vi "f.vi"() -> ()   [LabVIEW 2018]
uses:
  <vilib>/regexp/Match Regular Expression.xnode
panel:
  out "Array":string[](array[string])
  in  "length (rest) 2":i32
  in  "offset (0) 2":i32
  out "substring 2":string
  in  "length (rest)":i32
  in  "offset (0)":i32
  out "substring":string
  in  "Stop":bool
  out "Input":string
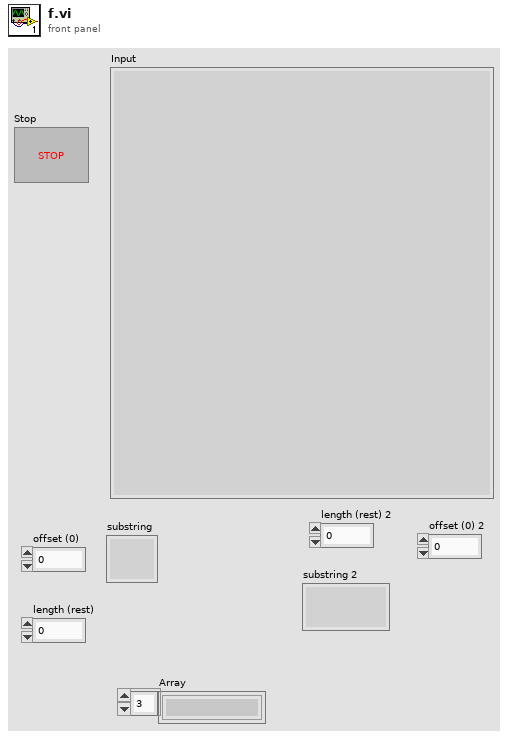
[diagram p1: front panel]
types:
  T1 = enum16{"open", "replace", "create", "open or create", "replace or create", "replace or create with confirmation"}
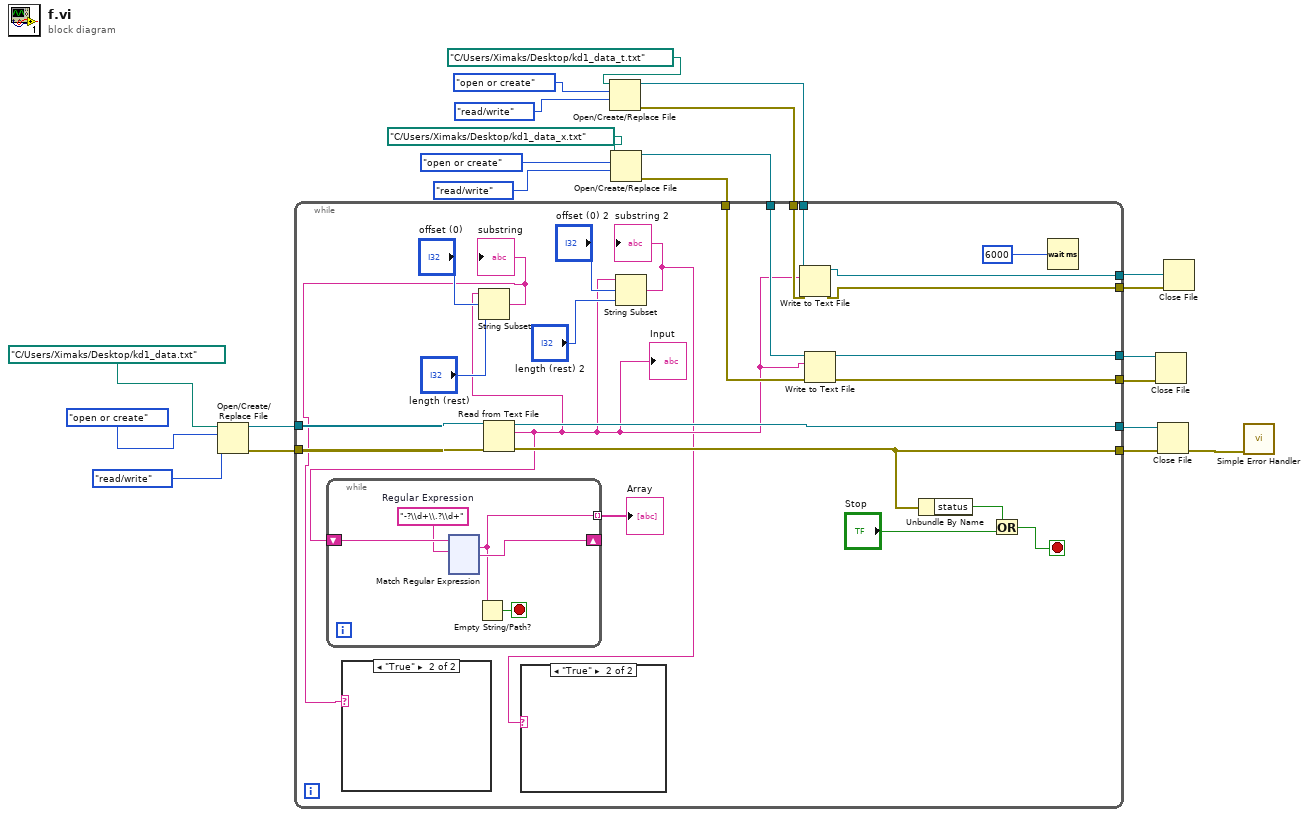
[diagram p0: block diagram]
diagram:
  n1 = Open/Create/Replace File(file path (use dialog)=path "C:/Users/Ximaks/Desktop/kd1_data.txt", operation (0:open)=T1."open or create", access (0:read/write)=enum16{"read/write", "read-only", "write-only"}."read/write") -> (refnum out=w22:refnum<file>, error out=w15:errorcluster)  [unwired: 3 in, 1 out]
  n2 = Open/Create/Replace File(file path (use dialog)=path "C:/Users/Ximaks/Desktop/kd1_data_t.txt", operation (0:open)=T1."open or create", access (0:read/write)=enum16{"read/write", "read-only", "write-only"}."read/write") -> (refnum out=w5:refnum<file>, error out=w6:errorcluster)  [unwired: 3 in, 1 out]
  n3 = Open/Create/Replace File(file path (use dialog)=path "C:/Users/Ximaks/Desktop/kd1_data_x.txt", operation (0:open)=T1."open or create", access (0:read/write)=enum16{"read/write", "read-only", "write-only"}."read/write") -> (refnum out=w7:refnum<file>, error out=w8:errorcluster)  [unwired: 3 in, 1 out]
  n4 = while {
    tunnel: w22 -> [w39]
    tunnel: w15 -> [w46]
    tunnel: [w40] -> w19
    tunnel: [w41] -> w18
    tunnel: w8 -> [w38]
    tunnel: w7 -> [w37]
    tunnel: w6 -> [w36]
    tunnel: w5 -> [w35]
    tunnel: [w34] -> w4
    tunnel: [w33] -> w3
    tunnel: [w32] -> w2
    tunnel: [w31] -> w1
    stop <- w44 stop-if-true
    n5 = Read from Text File(file (use dialog)=w39, error in=w46) -> (refnum out=w40:refnum<file>, text=w26:string, error out=w41:errorcluster)  [unwired: 2 in, 1 out]
    "Input" <- w26
    n6 = while {
      shift-right: [w50] -> _
      shift-left: w26 -> [w51]
      tunnel: [w48] -> w25 mode=indexing
      stop <- w47 stop-if-true
      w49 = "-?\\d+\\.?\\d+"  # Regular Expression
      n7 = xnode "Match Regular Expression"("input string"=w51, "regular expression"=w49) -> ("whole match"=w48:string, "after match"=w50:string)  [unwired: 4 in, 3 out]
      n8 = Empty String/Path?(string/path=w48) -> (empty?=w47:bool)
    }
    "Array" <- w25
    n9 = String Subset(string=w26, offset (0)="offset (0)", length (rest)="length (rest)") -> (substring=w24:string)
    "substring" <- w24
    n10 = case shown="\"True\"" w24 {
      frame "False", Default {
      }
      frame "True" {
      }
    }
    n11 = String Subset(string=w26, offset (0)="offset (0) 2", length (rest)="length (rest) 2") -> (substring=w23:string)
    "substring 2" <- w23
    n12 = case shown="\"True\"" w23 {
      frame "False", Default {
      }
      frame "True" {
      }
    }
    n13 = Write to Text File(file (use dialog)=w35, text=w26, error in=w36) -> (refnum out=w33:refnum<file>, error out=w34:errorcluster)  [unwired: 1 in, 1 out]
    n14 = Write to Text File(file (use dialog)=w37, text=w26, error in=w38) -> (refnum out=w32:refnum<file>, error out=w31:errorcluster)  [unwired: 1 in, 1 out]
    n15 = Unbundle By Name(w41) -> ("status"=w42:bool)
    n16 = Or(x=w42, y="Stop") -> (x .or. y?=w44:bool)
    n17 = Wait (ms)(milliseconds to wait=6000) -> ()  [unwired: 1 out]
  }
  n18 = Close File(refnum=w2, error in=w1) -> ()  [unwired: 2 out]
  n19 = Close File(refnum=w19, error in=w18) -> (error out=w17:errorcluster)  [unwired: 1 out]
  n20 = Close File(refnum=w3, error in=w4) -> ()  [unwired: 2 out]
  n21 = call <vilib>:"Simple Error Handler.vi"("error in (no error)"=w17) -> ()  [unwired: 4 in, 5 out]
